vi "MuxCardSwitch.vi"(6 "Single Needle":bool=TRUE, 7 "Probe Card Channels":i32=1, 8 "error in (no error)":errorcluster, 9 "disabled channels":u32[](array[numeric]), 10 "Switch to channel":i32, 11 "Pickering in":refnum<class "PickeringPrague.lvclass">) -> (0 "error out":errorcluster, 2 "last channel no.":i32, 3 "Pickering out":refnum<class "PickeringPrague.lvclass">)   [LabVIEW 2018, in "PickeringPrague.lvclass"]
uses:
  PickeringPrague.lvclass
panel:
  out "Display Matrix":bool[][](array[boolean])
  # "Pickering Multiplexer Settings"
  # "X1"
  # "X2"
  # "X3"
  # "X4"
  # "X5"
  # "X6"
  # "X7"
  # "X8"
  # "Y1  Y2  Y3  Y4"
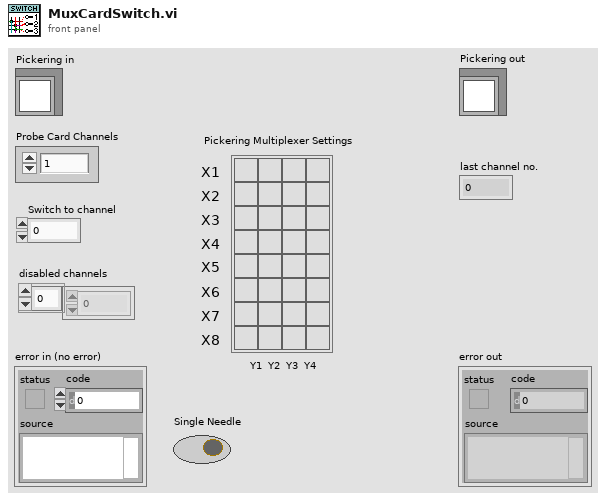
[diagram p1: front panel]
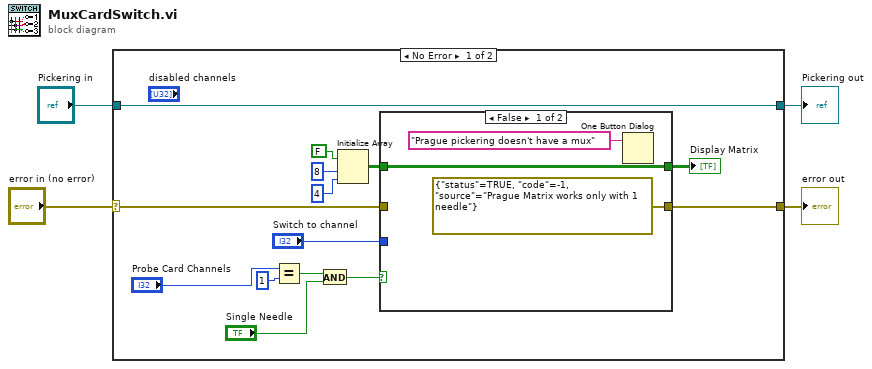
[diagram p0: block diagram]
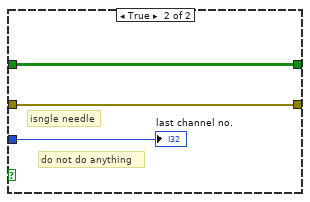
[diagram p2: hidden frame]
diagram:
  n1 = case shown="No Error" "error in (no error)" {
    selector: "error in (no error)" -> [w6 w26]
    tunnel: [w10 w26] -> w3
    tunnel: [w9 w25] -> w2
    tunnel: "Pickering in" -> [w9 w25]
    frame No Error {
      n2 = Equal?(x="Probe Card Channels", y=1) -> (x = y?=w12:bool)
      n3 = And(x=w12, y="Single Needle") -> (x .and. y?=w11:bool)
      n4 = Initialize Array(FALSE, 8, 4) -> (w7:bool[][])
      n5 = case shown="False" w11 {
        tunnel: [errorcluster {"status"=TRUE, "code"=-1, "source"="Prague Matrix works only with 1 needle"} ("error out") w23] -> w10
        tunnel: [w20 w24] -> w8
        tunnel: w7 -> [w20 w24]
        tunnel: w6 -> [_ w23]
        tunnel: "Switch to channel" -> [_ w22]
        frame False {
          n6 = One Button Dialog(message="Prague pickering doesn't have a mux") -> ()  [unwired: 1 in, 1 out]
        }
        frame True {
          # "do not do anything"
          # "isngle needle"
          "last channel no." <- w22
        }
      }
      "Display Matrix" <- w8
    }
    frame Error {
    }
  }
  "error out" <- w3
  "Pickering out" <- w2
